vi "Send Fetch Room Details.vi"(7 "Message Priority (Normal)":T1=enum."Normal", 8 "error in (no error)":errorcluster, 9 "Room No":string, 10 "Rooms Manager GUID":string, 11 "Message Enqueuer":refnum<class "Message Enqueuer.lvclass">) -> (0 "error out":errorcluster, 3 "Message Enqueuer out":refnum<class "Message Enqueuer.lvclass">)   [LabVIEW 2023, in "Incoming Hotel Management Tool Model Interface.lvlib" / "Fetch Room Details Msg.lvclass"]
doc: "This VI sends the message to an actor."
uses:
  Fetch Room Details Msg.lvclass
  Fetch Room Details Msg.lvclass/Fetch Room Details Msg.ctl
  <vilib>/ActorFramework/Message Enqueuer/Message Enqueuer.lvclass
  C:/Program Files/National Instruments/LabVIEW 2023/vi.lib/ActorFramework/Message/Message.lvclass
  C:/Users/bhaghyaraj/Trainings/NI Actor Framework/SDLC/Interfaces/Incoming Hotel Management Tool Model Interface Messages/Fetch Room Details Msg/Fetch Room Details Msg.lvclass
  <vilib>/ActorFramework/Message Enqueuer/Message Priority.ctl
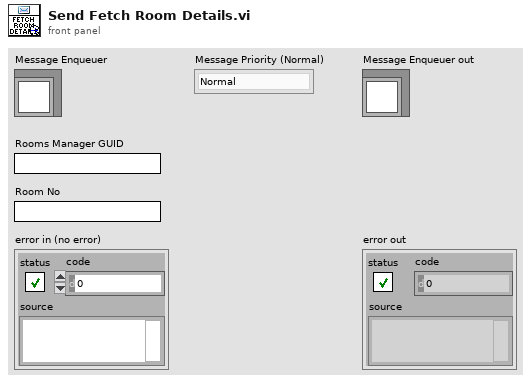
[diagram p1: front panel]
types:
  T1 = typedef "Actor Framework.lvlib/Message Enqueuer.lvclass/Message Priority.ctl" = enum16{"Low", "Normal", "High"}
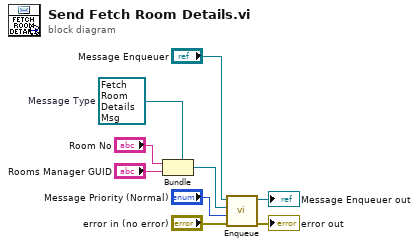
[diagram p0: block diagram]
diagram:
  w6 = refnum<class "Fetch Room Details Msg.lvclass"> refnum  # Message Type
  n1 = Bundle(cluster=w6, "Room No", "Rooms Manager GUID") -> (w5:refnum<class "Fetch Room Details Msg.lvclass">)
  n2 = call <vilib>:"Enqueue.vi"("error in (no error)"="error in (no error)", "Message Priority (Normal)"="Message Priority (Normal)", "Message"=w5, "Message Enqueuer in"="Message Enqueuer") -> ("error out"=→"error out":errorcluster, "Message Enqueuer out"=→"Message Enqueuer out":refnum<class "Message Enqueuer.lvclass">)  [unwired: 6 in]
